vi "Init Message Transport Singleton.vi"(8 "error in (no error)":errorcluster, 11 "Unique? (T)":bool=TRUE) -> (0 "error out":errorcluster, 3 "Message Transport Singleton out":refnum<class "Message Transport Singleton.lvclass">)   [LabVIEW 2016, in "Stream Mediator.lvlib" / "Message Transport Singleton.lvclass"]
doc: "--\nCopyright © 2017 Composed SystemsI All rights reserved.\n\nAuthor: Jon McBee <jon.mcbee@composed.io>\n\nThis library is provided \"AS IS\" ,WITHOUT WARRANTIES OR\nCONDITIONS OF ANY KIND, either express or implied.\n\nComposed Systems -- composed.io\n\nStream 0.0.1.1\nJon McBee - Composed Systems\nCopyright (c) 2017, Composed Systems"
uses:
  <userlib>/Composed Systems/Stream/Mediator/Classes/Message Transport Singleton/Message Transport Singleton.lvclass
  <userlib>/Composed Systems/Stream/Mediator/Classes/Message Interface/Message Interface.lvclass
  <userlib>/Composed Systems/Stream/Mediator/Classes/Message Transport Singleton/Message Transport Singleton.lvclass/Message Transport Singleton.ctl
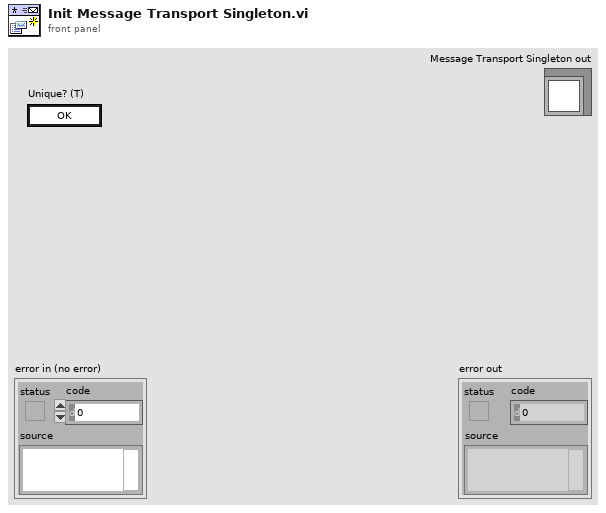
[diagram p1: front panel]
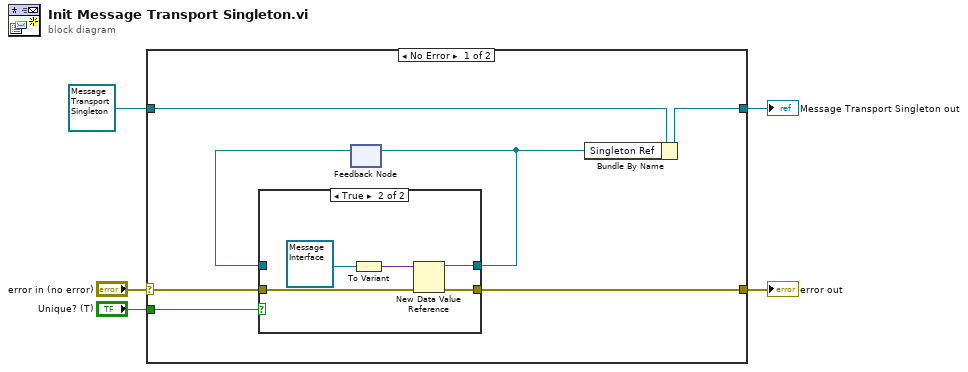
[diagram p0: block diagram]
diagram:
  n1 = case shown="No Error" "error in (no error)" {
    selector: "error in (no error)" -> [w12 w21]
    tunnel: [w11 w21] -> w4
    tunnel: [w8 w20] -> w2
    tunnel: refnum<class "Message Transport Singleton.lvclass"> refnum ("Message Transport Singleton in") -> [w9 w20]
    tunnel: "Unique? (T)" -> [w6 _]
    frame No Error {
      n2 = feedback #1() -> (w10:refnum<data-value>)  [unwired: 1 in]
      n3 = case shown="True" w6 {
        tunnel: w12 -> [w13 w16]
        tunnel: [w13 w15] -> w11
        tunnel: [w14 w17] -> w7
        tunnel: w10 -> [w14 _]
        frame False {
        }
        frame True {
          n4 = To Variant(anything=refnum<class "Message Interface.lvclass"> refnum ("Stream Mediator.lvlib:Message Interface.lvclass")) -> (Variant=w18:variant)
          n5 = New Data Value Reference(data value=w18, error in=w16) -> (data value reference=w17:refnum<data-value>, error out=w15:errorcluster)
        }
      }
      n6 = feedback-in #1(w7) -> ()
      n7 = Bundle By Name(cluster=w9, "Singleton Ref"=w7) -> (w8:refnum<class "Message Transport Singleton.lvclass">)
    }
    frame Error {
    }
  }
  "error out" <- w4
  "Message Transport Singleton out" <- w2
